vi "send&receive_multy_arrs.vi"() -> ()   [LabVIEW 2018, in "LV-0mq-Julia_roundtrip-lib.lvlib" / "LV2Julia_core.lvlib"]
uses:
  LV2Julia_core.lvlib
  Commands.ctl
  commands LV2Jl.ctl
  Server or client state.ctl
  d2cb43a9-9305-42fb-ad58-bce983510195.vi
  0f3c6ff9-6efb-4048-9743-f0faf74ba571.vi
  5398bb44-7854-4704-a5a4-70900ab1788b.vi
  1180a24e-9cfc-4814-956e-56f85e4fc15d.vi
  4837e4b1-53a7-49b6-9aef-263877b89a45.vi
  <vilib>/addons/zeromq/zmq_socket.lvclass
  StackFrame.ctl
  detailed error info.ctl
panel:
  out "U64arr":u64[](array[numeric])
  out "arrays equal":bool
  out "elems equal":bool
  in  "next":bool
  in  "stop LV only":bool
  in  "stop":bool
  out "detailed error info":T1
  out "elem sent":sgl
  out "elem received":dbl
  out "testarr":sgl[][](array[numeric])
  in  "index to return":cluster{"idx":u16[]}={"idx"=[3, 4, 1]} {"idx" min=1}
  out "Jl Server state out":T3
  out "short err code":u8
  out "final error":errorcluster
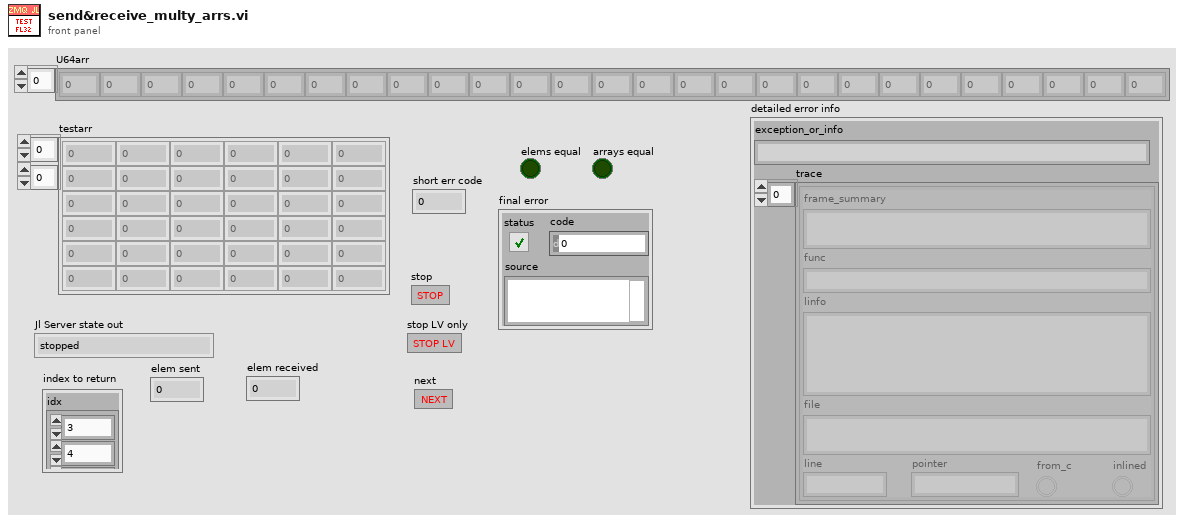
[diagram p1: front panel]
types:
  T1 = typedef "LV-0mq-Julia_roundtrip-lib.lvlib/detailed error info.ctl" = cluster{"exception_or_info":string, "trace":T2[]}
  T2 = typedef "LV-0mq-Julia_roundtrip-lib.lvlib/StackFrame.ctl" = cluster{"frame_summary":string, "func":string, "linfo":string, "file":string, "line":i32, "pointer":u64, "from_c":bool, "inlined":bool}
  T3 = typedef "LV-0mq-Julia_roundtrip-lib.lvlib/Server or client state.ctl" = enum16{"stopped", "running", "unknown"}
  T4 = typedef "LV-0mq-Julia_roundtrip-lib.lvlib/Commands.ctl" = enum16{"Start Jl-server & Init LV-client", "Send request & Get response ", "Stop Jl-server & Cleanup LV-client", "Cleanup LV-client", "Start Jl-server", "Stop Jl-server", "Init LV-Client", "Cleanup LV-Client", "(not allowed)", "Set LV Client state", "Set Jl Server state", "set ZMQ timeout", "read ZMQ timeout", "read-out state"}
  T5 = typedef "LV-0mq-Julia_roundtrip-lib.lvlib/commands LV2Jl.ctl" = u8
  T6 = typedef "LV-0mq-Julia_roundtrip-lib.lvlib/Bindata&description.ctl" = cluster{"bindata_descr":T7[], "bindata":u8[]}
  T7 = typedef "LV-0mq-Julia_roundtrip-lib.lvlib/Bindata description.ctl" = cluster{"nofbytes":i32, "numtype":string, "start":i32, "arrdims":i32[], "kwarg_name":string, "category":string}
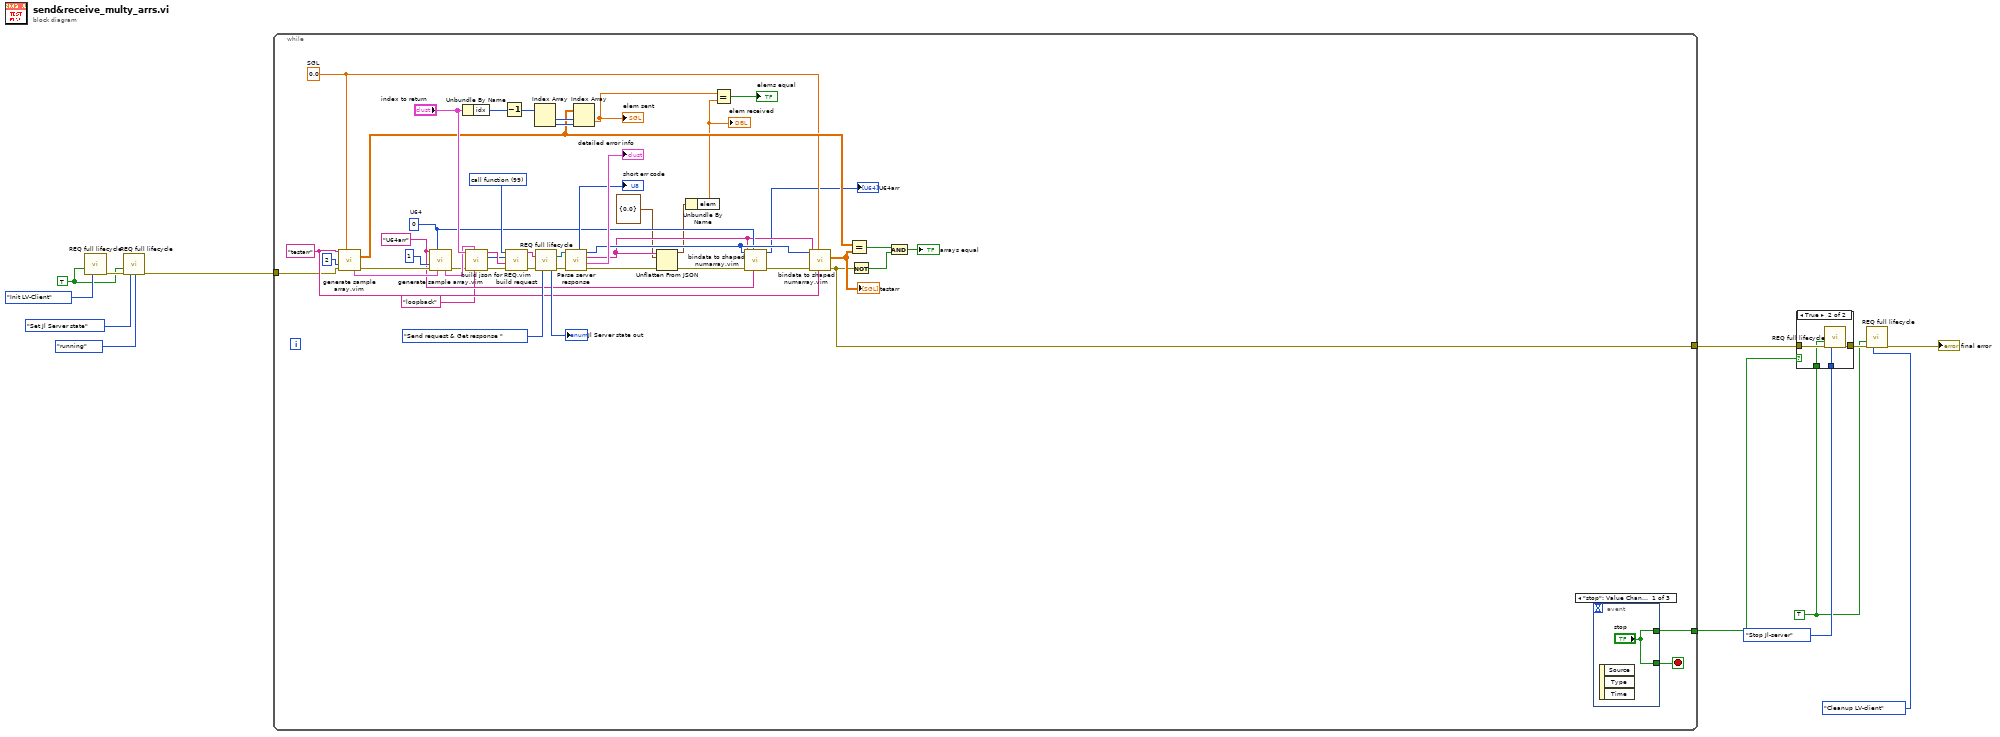
[diagram p0: block diagram]
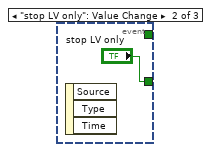
[diagram p2: hidden frame]
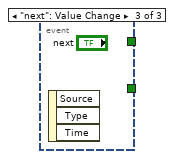
[diagram p3: hidden frame]
diagram:
  w4 = TRUE ("Force command")
  w8 = TRUE ("Force command")
  n1 = call "REQ full lifecycle.vi"("Force command"=w4, "command"=Commands."Init LV-Client") -> ("error out"=w6:errorcluster)  [unwired: 7 in, 6 out]
  n2 = call "REQ full lifecycle.vi"("Force command"=w4, "error in"=w6, "command"=Commands."Set Jl Server state", "Jl Server state in"=Server_or_client_state."running") -> ("error out"=w2:errorcluster)  [unwired: 5 in, 6 out]
  n3 = while {
    tunnel: w2 -> [w41]
    tunnel: [w33] -> w13
    tunnel: [w36] -> w1
    stop <- w37 stop-if-true
    w20 = "U64arr" ("kwarg_name")
    w22 = u64 0  # U64
    w30 = sgl 0.0  # SGL
    w48 = "testarr" ("Tag")
    w55 = T5 99 items=["call function"=99, "ping"=112, "stop"=115] ("Command")
    n4 = call "generate sample array.vim"("kwarg_name"=w48, "type"=w30, "dims"=2 ("arr1 dimension"), "error in (no error)"=w41) -> ("Array 2D"=w32:sgl[][], "Bindata & descr out"=w29:T6, "error out"=w27:errorcluster)  [unwired: 5 in, 4 out]
    n5 = call "generate sample array.vim"("kwarg_name"=w20, "type"=w22, "dims"=u8 1, "error in (no error)"=w27, "Bindata & descr in"=w29) -> ("Bindata & descr out"=w28:T6, "error out"=w26:errorcluster)  [unwired: 4 in, 5 out]
    n6 = Unbundle By Name("index to return") -> ("idx"=w45:u16[])
    n7 = call "build json for REQ.vim"("fun2call"="loopback", "Bindata & descr in"=w28, "error in (no error)"=w26, "Arguments 1"="index to return") -> ("error out"=w60:errorcluster, "bindata out"=w50:u8[], "JSON string out"=w51:string)  [unwired: 5 in]
    n8 = Decrement(x=w45) -> (x-1=w44:u16[])
    n9 = call "build request.vi"("error in (no error)"=w60, "JSON data"=w51, "binary data"=w50, "Command"=w55) -> ("error out"=w58:errorcluster, "REQ string"=w59:string)  [unwired: 6 in]
    n10 = Index Array(array=w44) -> (element #1=w39:u16, element #2=w38:u16)  [unwired: 2 in]
    n11 = call "REQ full lifecycle.vi"("data to send"=w59, "error in"=w58, "command"=Commands."Send request & Get response ") -> ("socket out"=w53:refnum<class "zmq_socket.lvclass">, "Jl Server state out"=→"Jl Server state out":T3, "error out"=w57:errorcluster)  [unwired: 6 in, 4 out]
    n12 = call "Parse server response.vi"("error in (no error)"=w57, "server response in"=w53) -> ("error out"=w46:errorcluster, "detailed error info"=→"detailed error info":T1, "JSON out"=w21:string, "binary data"=w25:u8[], "return code"=→"short err code":u8)  [unwired: 2 in, 3 out]
    n13 = Index Array(array=w32, index (row)=w39, index (col)=w38) -> (element=w43:sgl)
    "elem sent" <- w43
    n14 = Unflatten From JSON(JSON string=w21, type and defaults=cluster{"elem":dbl} {"elem"=0.0} ("parsed response"), error in (no error)=w46) -> (value=w16:cluster{"elem":dbl}, error out=w18:errorcluster)  [unwired: 4 in]
    n15 = Unbundle By Name(w16) -> ("elem"=w15:dbl)
    "elem received" <- w15
    n16 = Equal?(x=w43, y=w15) -> (x = y?=→"elems equal":bool)
    n17 = call "bindata to shaped numarray.vim"("name"=w20, "data type"=w22, "error in (no error)"=w18, "binary data"=w21, "JSON in"=w25) -> ("error out"=w24:errorcluster, "numarray 1D"=→"U64arr":u64[])  [unwired: 3 in, 2 out]
    n18 = call "bindata to shaped numarray.vim"("name"=w48, "data type"=w30, "error in (no error)"=w24, "binary data"=w21, "JSON in"=w25) -> ("error out"=w33:errorcluster, "numarray 2D"=w47:sgl[][])  [unwired: 3 in, 2 out]
    "testarr" <- w47
    n19 = Equal?(x=w32, y=w47) -> (x = y?=w34:bool)
    n20 = Not(x=w33) -> (.not. x?=w35:bool)
    n21 = And(x=w34, y=w35) -> (x .and. y?=→"arrays equal":bool)
    n22 = event shown="[0] \"stop\": Value Change" {
      selector: _ -> [_ _ _]
      dyn-events: _ -> [_ _ _]
      timeout: _ -> [_ _ _]
      tunnel: ["stop" "stop LV only" _] -> w37
      tunnel: ["stop" _ _] -> w36
      event "stop": Value Change {
        n23 = event-data() -> ()  [unwired: 1 in, 3 out]
      }
      event "stop LV only": Value Change {
        n24 = event-data() -> ()  [unwired: 1 in, 3 out]
      }
      event "next": Value Change {
        n25 = event-data() -> ()  [unwired: 1 in, 3 out]
      }
    }
  }
  n26 = case shown="True" w1 {
    tunnel: w13 -> [w64 w68]
    tunnel: Commands."Stop Jl-server" ("command") -> [_ w67]
    tunnel: [w64 w66] -> w11
    tunnel: w8 -> [_ w65]
    frame False {
    }
    frame True {
      n27 = call "REQ full lifecycle.vi"("Force command"=w65, "error in"=w68, "command"=w67) -> ("error out"=w66:errorcluster)  [unwired: 6 in, 6 out]
    }
  }
  n28 = call "REQ full lifecycle.vi"("Force command"=w8, "error in"=w11, "command"=Commands."Cleanup LV-client") -> ("error out"=→"final error":errorcluster)  [unwired: 6 in, 6 out]
